vi "PNG Picture Size Reader.vi"(8 "error in (no error)":errorcluster, 11 "Graphic":path) -> (0 "error out":errorcluster, 1 "pic height":i16, 2 "pic width":i16, 3 "custom image":T1)   [LabVIEW 2021, in "Pop-Up.lvlib" / "PNG Parent.lvclass"]
doc: "get the information for the size of the custom image and the background info\n\n<b>Code Developed By:</b> +\nDaniel Coons +\nhttps://github.com/danielcoons/tsc-pop-up"
uses:
  PNG Parent.lvclass
  <vilib>/picture/picture.llb/imagedata.ctl
  PNG Parent.lvclass/PNG Parent.ctl
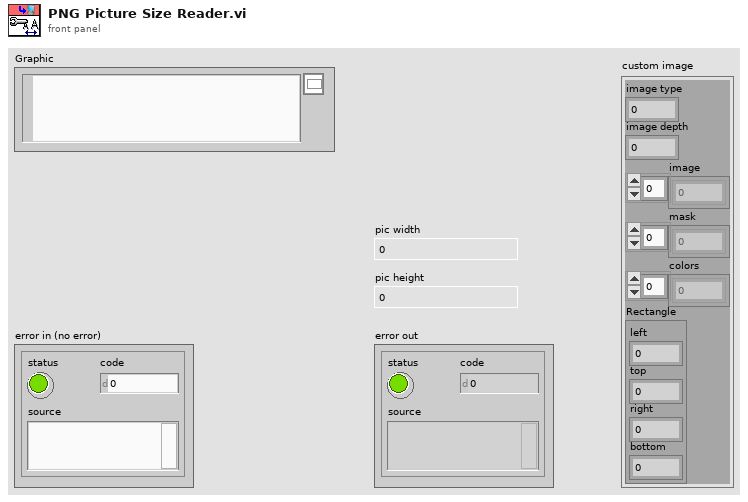
[diagram p1: front panel]
types:
  T1 = typedef "imagedata.ctl" = cluster{"image type":i32, "image depth":i32, "image":u8[], "mask":u8[], "colors":u32[], "Rectangle":cluster{"left":i16, "top":i16, "right":i16, "bottom":i16}}
  T2 = cluster{"left":i16, "top":i16, "right":i16, "bottom":i16}
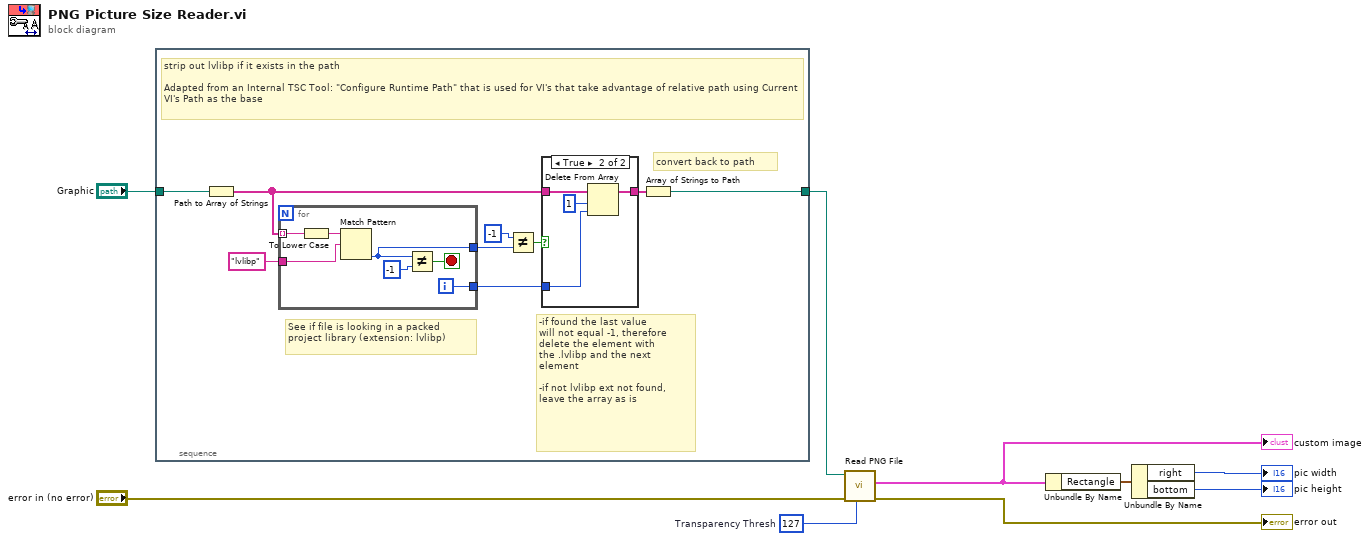
[diagram p0: block diagram]
diagram:
  w1 = u8 127  # Transparency Thresh
  n1 = stacked-sequence {
    tunnel: [w10] -> w2
    tunnel: "Graphic" -> [w11]
    frame #0 {
      # "convert back to path"
      # "-if found the last value\nwill not equal -1, therefore\ndelete the element with\nthe .lvlibp and the next\nelement\n\n-if not lvlibp ext not found,\nleave the array as is"
      # "See if file is looking in a packed\nproject library (extension: lvlibp)"
      # "strip out lvlibp if it exists in the path\n\nAdapted from an Internal TSC Tool: \"Configure Runtime Path\" that is used for VI's that take advantage of relative path using Current VI's Path as the base"
      n2 = Path to Array of Strings(0:w11) -> (2:w17:string[])  [unwired: 1 out]
      n3 = for {
        tunnel: w17 -> [w30] mode=indexing
        tunnel: "lvlibp" ("element") -> [w28]
        tunnel: [w27] -> w16
        tunnel: [w24] -> w15
        i -> [w27]
        stop <- w25 stop-if-true
        n4 = To Lower Case(string=w30) -> (all lower case string=w29:string)
        n5 = Match Pattern(string=w29, regular expression=w28) -> (offset past match=w24:i32)  [unwired: 1 in, 3 out]
        n6 = Not Equal?(x=w24, y=-1) -> (x != y?=w25:bool)
      }
      n7 = Not Equal?(x=-1 ("y"), y=w15) -> (x != y?=w13:bool)
      n8 = case shown="True" w13 {
        tunnel: w17 -> [w19 w23]
        tunnel: w16 -> [_ w22]
        tunnel: [w19 w20] -> w12
        frame False {
        }
        frame True {
          n9 = Delete From Array(array=w23, length=1, index=w22) -> (array with subset deleted=w20:string[])  [unwired: 1 out]
        }
      }
      n10 = Array of Strings to Path(0:w12) -> (2:w10:path)  [unwired: 1 in]
    }
  }
  n11 = call <vilib>:"Read PNG File.vi"("Transparency Thresh"=w1, "error in (no error)"="error in (no error)", "path to PNG file"=w2) -> ("error out"=→"error out":errorcluster, "image data"=w5:T1)  [unwired: 6 in, 1 out]
  "custom image" <- w5
  n12 = Unbundle By Name(w5) -> ("Rectangle"=w6:T2)
  n13 = Unbundle By Name(w6) -> ("right"=→"pic width":i16, "bottom"=→"pic height":i16)
